vi "Cross_spectra.vi"(4 "block number":i32, 5 "S11 input array":dbl[](array[numeric]) format="%.2f", 6 "sampling frequency":dbl format="%.2f", 7 "S22 input array":dbl[](array[numeric]) format="%.2f", 8 "Im(S12) input array":dbl[](array[numeric]) format="%.2f", 9 "Re(S12) input array":dbl[](array[numeric]) format="%.2f", 10 "U2":dbl[](array[numeric]) format="%.2f", 11 "U1":dbl[](array[numeric]) format="%.2f") -> (0 "Im(S12) output array":dbl[](array[numeric]) format="%.2f", 1 "Re(S12) output array":dbl[](array[numeric]) format="%.2f", 2 "Phase array":dbl[](array[numeric]) format="%.2f", 3 "Coherence array":dbl[](array[numeric]) format="%.2f")   [LabVIEW 2010]
uses:
  <vilib>/Analysis/2dsp.llb/Cross Power (DBL).vi
  <vilib>/Analysis/NI_AALBase.lvlib
  <vilib>/Analysis/NI_AALPro.lvlib
panel:
  out "error":i32
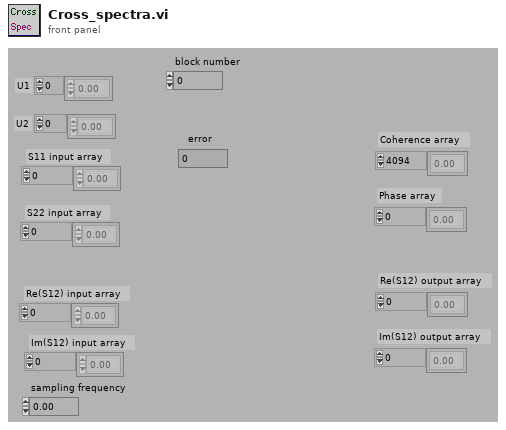
[diagram p1: front panel]
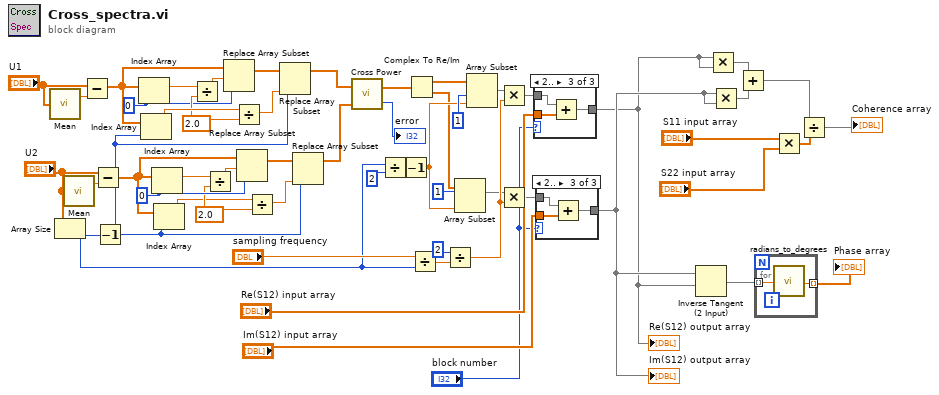
[diagram p0: block diagram]
diagram:
  w11 = 2.0
  w12 = 0
  w22 = 0
  w23 = 2.0
  n1 = call <vilib>:"Mean.vi"("X"="U1") -> ("mean"=w55:dbl)  [unwired: 1 out]
  n2 = Array Size(array="U2") -> (size(s)=w16:i32)
  n3 = call <vilib>:"Mean.vi"("X"="U2") -> ("mean"=w54:dbl)  [unwired: 1 out]
  n4 = Subtract(x="U1", y=w55) -> (x-y=w19:dbl[])
  n5 = Subtract(x="U2", y=w54) -> (x-y=w7:dbl[])
  n6 = Decrement(x=w16) -> (x-1=w6:i32)
  n7 = Index Array(array=w19, index=w22) -> (element=w25:dbl)
  n8 = Index Array(array=w19, index=w6) -> (element=w24:dbl)
  n9 = Index Array(array=w7, index=w12) -> (element=w9:dbl)
  n10 = Index Array(array=w7, index=w6) -> (element=w10:dbl)
  n11 = Divide(x=w25, y=w23) -> (x/y=w21:dbl)
  n12 = Divide(x=w9, y=w11) -> (x/y=w13:dbl)
  n13 = Replace Array Subset(array=w19, new element=w21, index=w22) -> (w26:dbl[])
  n14 = Divide(x=w24, y=w23) -> (x/y=w20:dbl)
  n15 = Replace Array Subset(array=w7, new element=w13, index=w12) -> (w8:dbl[])
  n16 = Divide(x=w10, y=w11) -> (x/y=w14:dbl)
  n17 = Replace Array Subset(array=w26, new element=w20, index=w6) -> (w18:dbl[])
  n18 = Replace Array Subset(array=w8, new element=w14, index=w6) -> (w15:dbl[])
  n19 = call-poly <vilib>:"Cross Power.vi"("Y"=w15, "X"=w18) -> ("error"=→"error":i32, "Sxy"=w38:cdb[])
  n20 = Divide(x=w16, y=2) -> (x/y=w46:dbl)
  n21 = Decrement(x=w46) -> (x-1=w45:dbl)
  n22 = Complex To Re/Im(x + iy=w38) -> (x=w37:dbl[], y=w36:dbl[])
  n23 = Divide(x="sampling frequency", y=w16) -> (x/y=w28:dbl)
  n24 = Divide(x=2, y=w28) -> (x/y=w41:dbl)
  n25 = Array Subset(array=w36, index=1, length=w45) -> (w40:dbl[])
  n26 = Array Subset(array=w37, index=1, length=w45) -> (w52:dbl[])
  n27 = Multiply(x=w52, y=w41) -> (x*y=w31:dbl[])
  n28 = Multiply(x=w40, y=w41) -> (x*y=w32:dbl[])
  n29 = case shown="2.." "block number" {
    tunnel: [w56 w57 w60] -> w4
    tunnel: w31 -> [w56 w57 w59]
    tunnel: "Re(S12) input array" -> [_ _ w58]
    frame ..0 {
    }
    frame 1 {
    }
    frame 2.. {
      n30 = Add(x=w59, y=w58) -> (x+y=w60:dbl[])
    }
  }
  "Re(S12) output array" <- w4
  n31 = case shown="2.." "block number" {
    tunnel: [w61 w62 w65] -> w5
    tunnel: w32 -> [w61 w62 w64]
    tunnel: "Im(S12) input array" -> [_ _ w63]
    frame ..0 {
    }
    frame 1 {
    }
    frame 2.. {
      n32 = Add(x=w64, y=w63) -> (x+y=w65:dbl[])
    }
  }
  "Im(S12) output array" <- w5
  n33 = Inverse Tangent (2 Input)(1:w4, 2:w5) -> (0:w3:dbl[])
  n34 = Multiply(x=w4, y=w4) -> (x*y=w35:dbl[])
  n35 = Multiply(x=w5, y=w5) -> (x*y=w34:dbl[])
  n36 = Add(x=w35, y=w34) -> (x+y=w33:dbl[])
  n37 = for {
    tunnel: w3 -> [w67] mode=indexing
    tunnel: [w66] -> w43 mode=indexing
    n38 = call "radians_to_degrees.vi"("radians"=w67) -> ("degrees"=w66:dbl)
  }
  "Phase array" <- w43
  n39 = Multiply(x="S11 input array", y="S22 input array") -> (x*y=w48:dbl[])
  n40 = Divide(x=w33, y=w48) -> (x/y=→"Coherence array":dbl[])
